vi "example test.vi"() -> ()   [LabVIEW 2013, in "UI reference module tests.lvlib"]
uses:
  UI reference module tests.lvlib
  module/execution/UI Reference runtime.lvclass
  module/configuration/UI Reference configuration.lvclass
  <vilib>/NI/Tag Bus/tag/tag descriptor.lvclass/tag descriptor.ctl
  <vilib>/NI/Tag Bus/tag/Data Type.ctl
  <vilib>/NI/Tag Bus/dictionary/data dictionary.lvclass/data dictionary.ctl
  <vilib>/NI/Tag Bus/dictionary/lookup polymorphs/locate double.vi
  <vilib>/NI/Tag Bus/dictionary/lookup polymorphs/locate Boolean.vi
  <vilib>/NI/Tag Bus/dictionary/lookup polymorphs/locate String.vi
  <vilib>/NI/Tag Bus/table/data polymorphs/read one/read Double.vi
  <vilib>/NI/Tag Bus/table/data polymorphs/write one/write Double.vi
  <vilib>/NI/Tag Bus/table/data polymorphs/read one/read Boolean.vi
  <vilib>/NI/Tag Bus/table/data polymorphs/write one/write Boolean.vi
  <vilib>/NI/Tag Bus/table/data polymorphs/read one/read String.vi
  <vilib>/NI/Tag Bus/table/data polymorphs/write one/write String.vi
  <vilib>/NI/Tag Bus/tag/read tag name.vi
  <vilib>/NI/Tag Bus/dictionary/search/find data index.vi
  <vilib>/NI/Tag Bus/dictionary/search/search string list.vi
  <vilib>/NI/Tag Bus/dictionary/tag not found.vi
  <vilib>/NI/Tag Bus/dictionary/data dictionary.lvclass
  <vilib>/NI/Tag Bus/table/data table.lvlib
  <vilib>/NI/Tag Bus/tag/tag descriptor.lvclass
panel:
  out "u8 out":u8
  out "exec settings":errorcluster
  in  "Stop wkaround":errorcluster
  out "String out":string
  in  "String in":string
  out "bool out":bool
  in  "bool in":bool
  out "dbl out":dbl
  in  "dbl in":dbl
  out "final error":errorcluster
  out "init error":errorcluster
  out "serialization problem":errorcluster
  out "invalid configuration":errorcluster
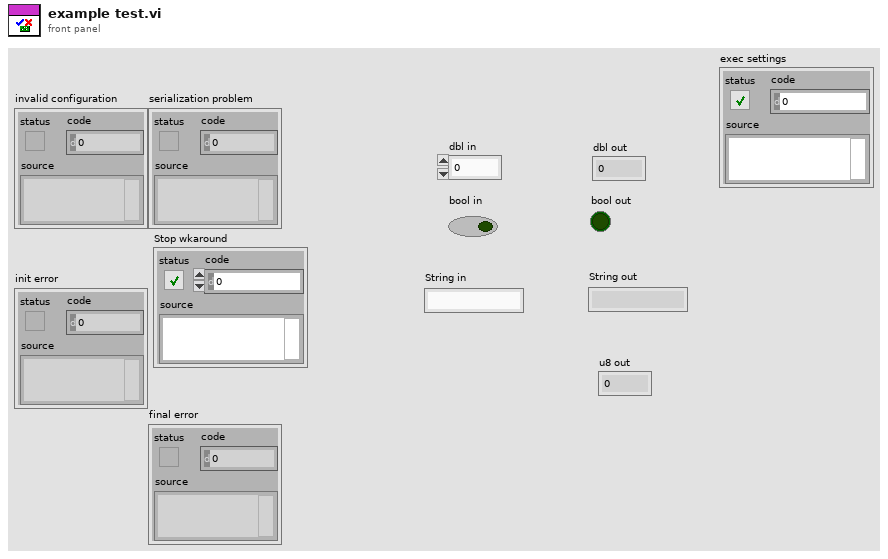
[diagram p1: front panel]
types:
  T1 = typedef "tag bus.lvlib/tag descriptor.lvclass/Data Type.ctl" = enum16{"Double", "Single", "I64", "I32", "I16", "I8", "U64", "U32", "U16", "U8", "Boolean", "String", "Array of Double", "Array of Single", "Array of I64", "Array of I32", "Array of I16", "Array of I8", "Array of U64", "Array of U32", "Array of U16", "Array of U8", "Array of Boolean", "Array of String"}
  T2 = typedef "TBM channel.lvclass/data tables.ctl" = cluster{"input data":T3, "processing parameter":T3, "processing result":T3, "output data":T3}
  T3 = typedef "tag bus.lvlib/dictionary table pair.ctl" = cluster{"data dictionary":refnum<class "data dictionary.lvclass">, "data table":T4}
  T4 = typedef "tag bus.lvlib/data table.lvlib/data table.ctl" = cluster{"Double":dbl[], "Single":sgl[], "I64":i64[], "I32":i32[], "I16":i16[], "I8":i8[], "U64":u64[], "U32":u32[], "U16":u16[], "U8":u8[], "Boolean":bool[], "String":string[], "Array of Double":cluster{"DBL Array":dbl[]}[], "Array of Single":cluster{"SGL Array":sgl[]}[], "Array of I64":cluster{"I64 Array":i64[]}[], "Array of I32":cluster{"I32 Array":i32[]}[], "Array of I16":cluster{"I16 Array":i16[]}[], "Array of I8":cluster{"I8 Array":i8[]}[], "Array of U64":cluster{"U64 Array":u64[]}[], "Array of U32":cluster{"U32 Array":u32[]}[], "Array of U16":cluster{"U16 Array":u16[]}[], "Array of U8":cluster{"U8 Array":u8[]}[], "Array of Boolean":cluster{"Boolean Array":bool[]}[], "Array of String":cluster{"String Array":string[]}[]}
  T5 = typedef "TBM module execution interface.lvclass/execution settings.ctl" = cluster{"reads inputs":bool, "processes data":bool, "writes outputs":bool}
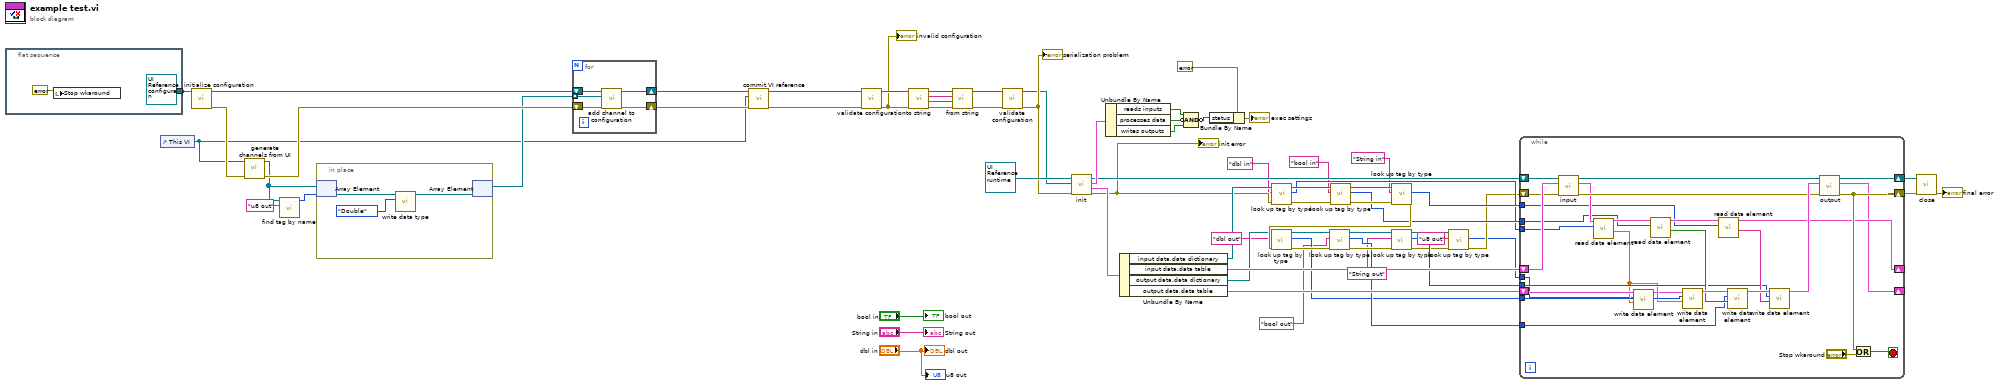
[diagram p0: block diagram]
diagram:
  n1 = flat-sequence {
    tunnel: [refnum<class "UI Reference configuration.lvclass"> refnum ("tag bus configurable plugin module configuration")] -> w50
    frame #0 {
      n2 = local write "Stop wkaround"(errorcluster {"status"=FALSE, "code"=0, "source"=""} ("Stop wkaround")) -> ()
    }
  }
  n3 = control-ref of="This VI"() -> (w1:refnum<vi>)
  n4 = call-dynamic "initialize configuration.vi"("configuration in"=w50) -> ("error out"=w48:errorcluster, "configuration out"=w46:refnum<class "UI Reference configuration.lvclass">)  [unwired: 8 in, 1 out]
  n5 = call "generate channels from UI.vi"("error in"=w48, "VI Refnum"=w1) -> ("error out"=w47:errorcluster, "channels"=w12:refnum<class "TBM channel.lvclass">[])  [unwired: 8 in]
  n6 = call <vilib>:"find tag by name.vi"("name"="u8 out", "tags in"=w12) -> ("index"=w11:i32)  [unwired: 9 in]
  n7 = in-place {
    n8 = in-place-array #1(w12, w11) -> (w75:refnum<class "TBM channel.lvclass">)
    n9 = call <vilib>:"write data type.vi"("data type"=Data_Type."Double", "system tag in"=w75) -> ("system tag out"=w74:refnum<class "TBM channel.lvclass">)  [unwired: 8 in, 1 out]
    n10 = in-place-array #1(w74) -> (w10:refnum<class "TBM channel.lvclass">[])  [unwired: 1 out]
  }
  n11 = for {
    shift-right: [w80] -> w3
    shift-left: w46 -> [w78]
    shift-right: [w79] -> w49
    shift-left: w47 -> [w77]
    tunnel: w10 -> [w76] mode=indexing
    n12 = call "add channel to configuration.vi"("error in"=w77, "channel"=w76, "UI Reference configuration in"=w78) -> ("error out"=w79:errorcluster, "UI Reference configuration out"=w80:refnum<class "UI Reference configuration.lvclass">)  [unwired: 7 in]
  }
  n13 = call "commit VI reference.vi"("error in"=w49, "VI Refnum in"=w1, "UI Reference configuration in"=w3) -> ("error out"=w4:errorcluster, "UI Reference configuration out"=w2:refnum<class "UI Reference configuration.lvclass">)  [unwired: 6 in, 1 out]
  n14 = call-dynamic "validate configuration.vi"("error in"=w4, "UI Reference configuration in"=w2) -> ("error out"=w69:errorcluster, "UI Reference configuration out"=w70:refnum<class "UI Reference configuration.lvclass">)  [unwired: 8 in]
  "invalid configuration" <- w69
  n15 = call-dynamic "to string.vi"("error in"=w69, "UI Reference configuration in"=w70) -> ("error out"=w65:errorcluster, "data"=w66:string, "version"=w67:string, "UI Reference configuration out"=w68:refnum<class "UI Reference configuration.lvclass">)  [unwired: 6 in]
  n16 = call-dynamic "from string.vi"("error in"=w65, "data"=w66, "version"=w67, "UI Reference configuration in"=w68) -> ("error out"=w63:errorcluster, "UI Reference configuration out"=w64:refnum<class "UI Reference configuration.lvclass">)  [unwired: 6 in]
  n17 = call-dynamic "validate configuration.vi"("error in"=w63, "UI Reference configuration in"=w64) -> ("error out"=w61:errorcluster, "UI Reference configuration out"=w60:refnum<class "UI Reference configuration.lvclass">)  [unwired: 8 in]
  "serialization problem" <- w61
  n18 = call-dynamic "init.vi"("error in"=w61, "UI Reference configuration in"=w60, "UI Reference runtime in"=refnum<class "UI Reference runtime.lvclass"> refnum ("tag bus configurable plugin module")) -> ("error out"=w32:errorcluster, "data allocations"=w55:T2, "execution settings"=w59:T5, "UI Reference runtime out"=w54:refnum<class "UI Reference runtime.lvclass">)  [unwired: 5 in]
  "init error" <- w32
  n19 = Unbundle By Name(w59) -> ("reads inputs"=w56:bool, "processes data"=w58:bool, "writes outputs"=w57:bool)
  n20 = Unbundle By Name(w55) -> ("input data.data dictionary"=w33:refnum<class "data dictionary.lvclass">, "input data.data table"=w44:T4, "output data.data dictionary"=w36:refnum<class "data dictionary.lvclass">, "output data.data table"=w45:T4)
  n21 = Compound Arithmetic op=AND(w56, invert w58, w57) -> (invert w18:bool)
  n22 = Bundle By Name(cluster=errorcluster {"status"=FALSE, "code"=0, "source"=""} ("error out"), "status"=w18) -> (→"exec settings":errorcluster)
  n23 = call-poly <vilib>:"look up tag by type.vi"("error in"=w32, "name"="dbl in", "data dictionary in"=w33) -> ("error out"=w42:errorcluster, "index"=w29:i32, "data dictionary out"=w43:refnum<class "data dictionary.lvclass">)  [unwired: 6 in]
  n24 = call-poly <vilib>:"look up tag by type.vi"("error in"=w42, "name"="bool in", "data dictionary in"=w43) -> ("error out"=w40:errorcluster, "index"=w30:i32, "data dictionary out"=w41:refnum<class "data dictionary.lvclass">)  [unwired: 6 in]
  n25 = call-poly <vilib>:"look up tag by type.vi"("error in"=w40, "name"="String in", "data dictionary in"=w41) -> ("error out"=w37:errorcluster, "index"=w31:i32)  [unwired: 6 in, 1 out]
  n26 = call-poly <vilib>:"look up tag by type.vi"("error in"=w37, "name"="dbl out", "data dictionary in"=w36) -> ("error out"=w38:errorcluster, "index"=w26:i32, "data dictionary out"=w35:refnum<class "data dictionary.lvclass">)  [unwired: 6 in]
  n27 = call-poly <vilib>:"look up tag by type.vi"("error in"=w38, "name"="bool out", "data dictionary in"=w35) -> ("error out"=w39:errorcluster, "index"=w27:i32, "data dictionary out"=w34:refnum<class "data dictionary.lvclass">)  [unwired: 6 in]
  n28 = call-poly <vilib>:"look up tag by type.vi"("error in"=w39, "name"="String out", "data dictionary in"=w34) -> ("error out"=w9:errorcluster, "index"=w28:i32, "data dictionary out"=w8:refnum<class "data dictionary.lvclass">)  [unwired: 6 in]
  n29 = call-poly <vilib>:"look up tag by type.vi"("error in"=w9, "name"="u8 out", "data dictionary in"=w8) -> ("error out"=w7:errorcluster, "index"=w6:i32)  [unwired: 6 in, 1 out]
  n30 = while {
    shift-right: [w95] -> w52
    shift-left: w7 -> [w97]
    shift-right: [w106] -> w53
    shift-left: w54 -> [w109]
    tunnel: w31 -> [w92]
    tunnel: w30 -> [w91]
    tunnel: w29 -> [w90]
    tunnel: w28 -> [w89]
    tunnel: w27 -> [w88]
    tunnel: w26 -> [w87]
    tunnel: w6 -> [w84]
    shift-right: [w82] -> _
    shift-left: w44 -> [w98]
    shift-right: [w81] -> _
    shift-left: w45 -> [w86]
    stop <- w93 stop-if-true
    n31 = call-dynamic "input.vi"("error in"=w97, "data table in"=w98, "UI Reference runtime in"=w109) -> ("error out"=w105:errorcluster, "data table out"=w96:T4, "UI Reference runtime out"=w108:refnum<class "UI Reference runtime.lvclass">)  [unwired: 6 in]
    n32 = call-poly <vilib>:"read data element.vi"("index"=w90, "data table in"=w96) -> ("value"=w85:dbl, "data table out"=w102:T4)  [unwired: 8 in]
    n33 = call-poly <vilib>:"write data element.vi"("value"=w85, "index"=w84, "data table in"=w86) -> ("data table out"=w83:T4)  [unwired: 8 in]
    n34 = call-poly <vilib>:"read data element.vi"("index"=w91, "data table in"=w102) -> ("value"=w99:bool, "data table out"=w101:T4)  [unwired: 8 in]
    n35 = call-poly <vilib>:"write data element.vi"("value"=w85, "index"=w87, "data table in"=w83) -> ("data table out"=w103:T4)  [unwired: 8 in]
    n36 = call-poly <vilib>:"read data element.vi"("index"=w92, "data table in"=w101) -> ("value"=w100:string, "data table out"=w82:T4)  [unwired: 8 in]
    n37 = call-poly <vilib>:"write data element.vi"("value"=w99, "index"=w88, "data table in"=w103) -> ("data table out"=w104:T4)  [unwired: 8 in]
    n38 = call-poly <vilib>:"write data element.vi"("value"=w100, "index"=w89, "data table in"=w104) -> ("data table out"=w107:T4)  [unwired: 8 in]
    n39 = call-dynamic "output.vi"("error in"=w105, "data table in"=w107, "UI Reference runtime in"=w108) -> ("error out"=w95:errorcluster, "data table out"=w81:T4, "UI Reference runtime out"=w106:refnum<class "UI Reference runtime.lvclass">)  [unwired: 6 in]
    n40 = Or(x=w95, y="Stop wkaround") -> (x .or. y?=w93:bool)
  }
  n41 = call-dynamic "close.vi"("error in"=w52, "UI Reference runtime in"=w53) -> ("error out"=→"final error":errorcluster)  [unwired: 9 in]
  "dbl out" <- "dbl in"
  "bool out" <- "bool in"
  "String out" <- "String in"
  "u8 out" <- "dbl in"
